vi "Get Relay State.vi"(8 "error in (no error)":errorcluster, 10 "SLSC Switch in":refnum<class "SLSC Switch.lvclass">, 11 "DevicePropertyRelay in":refnum<class "DevicePropertyRelay.lvclass">) -> (0 "error out":errorcluster, 1 "RelayPosition":T1=10 caption="position" items=["Open"=10, "Closed"=11], 2 "SLSC Switch out":refnum<class "SLSC Switch.lvclass">, 3 "DevicePropertyRelay out":refnum<class "DevicePropertyRelay.lvclass">)   [LabVIEW 2015, in "DevicePropertyRelay.lvclass"]
uses:
  DevicePropertyRelay.lvclass
  slscsl/RelayPosition.ctl
  SLSC Switch/SLSC Switch.lvclass
  SLSC Switch/SLSC Switch.lvclass/SLSC Switch.ctl
  DevicePropertyRelay.lvclass/DevicePropertyRelay.ctl
  <vilib>/SLSC/Get Device Property (Bool).vi
  <vilib>/SLSC/SLSC.lvlib
  slscsl/slscsl.lvclass
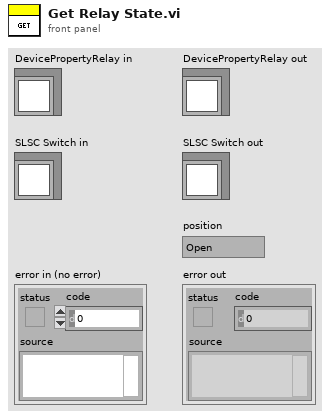
[diagram p1: front panel]
types:
  T1 = typedef "slscsl.lvclass/RelayPosition.ctl" = i32
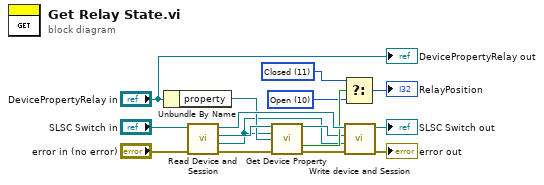
[diagram p0: block diagram]
diagram:
  w6 = T1 10 items=["Open"=10, "Closed"=11] ("f")
  w7 = T1 11 items=["Open"=10, "Closed"=11] ("RelayPosition")
  n1 = Unbundle By Name("DevicePropertyRelay in") -> ("property"=w9:refnum<k21>)
  n2 = call "Read Device and Session.vi"("error in (no error)"="error in (no error)", "SLSC Switch in"="SLSC Switch in") -> ("error out"=w2:errorcluster, "device"=w3:refnum<k21>, "session"=w10:refnum<k21>, "SLSC Switch out"=w14:refnum<class "SLSC Switch.lvclass">)  [unwired: 6 in]
  n3 = call-poly <vilib>:"Get Device Property.vi"("session in"=w10, "devices"=w3, "property"=w9, "error in (no error)"=w2) -> ("session out"=w4:refnum<k21>, "property value"=w8:bool, "error out"=w1:errorcluster)  [unwired: 9 in]
  n4 = Select(t=w7, s=w8, f=w6) -> (s? t:f=→"RelayPosition":T1)
  n5 = call "Write device and Session.vi"("error in (no error)"=w1, "device"=w3, "session"=w4, "SLSC Switch in"=w14) -> ("error out"=→"error out":errorcluster, "SLSC Switch out"=→"SLSC Switch out":refnum<class "SLSC Switch.lvclass">)  [unwired: 6 in]
  "DevicePropertyRelay out" <- "DevicePropertyRelay in"
